vi "Save.vi"(8 "error in (no error)":errorcluster, 9 "new command":string, 10 "Msg in":T1, 11 "FakePressureController in":refnum<class "Tapedrive_ESP301.lvclass">) -> (0 "error out":errorcluster, 1 "Path":path, 2 "Msg out":T1, 3 "FakePressureController out":refnum<class "Tapedrive_ESP301.lvclass">, 4 "new command":string)   [LabVIEW 2011, in "Tapedrive_ESP301.lvclass"]
uses:
  Tapedrive_ESP301.lvclass
  DriverMsg.ctl
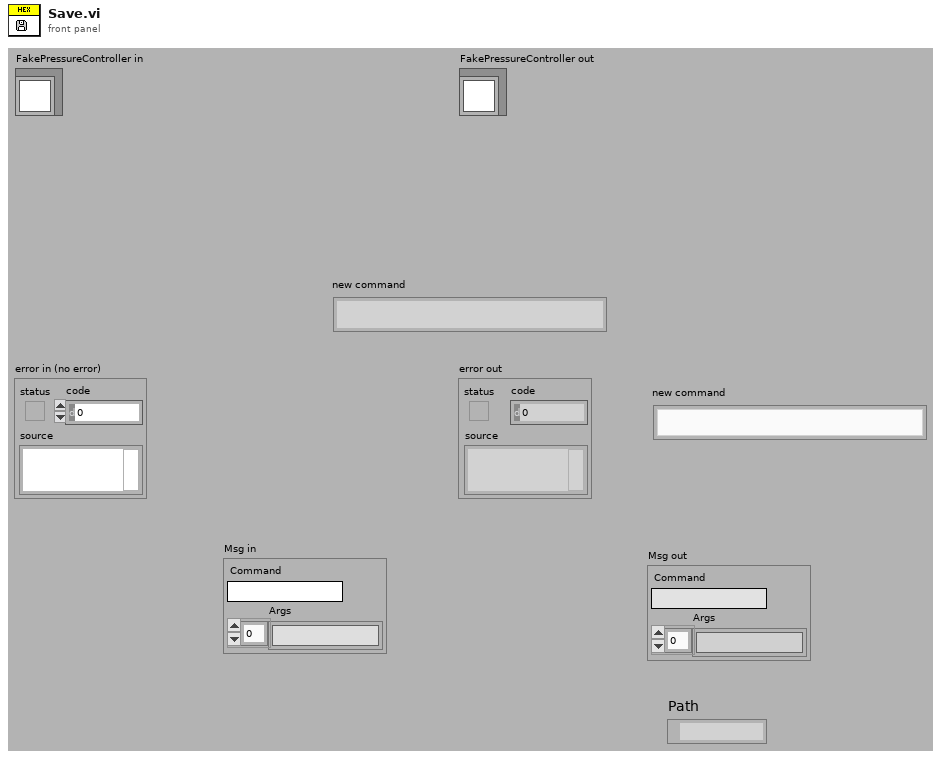
[diagram p1: front panel]
types:
  T1 = typedef "DriverMsg.ctl" = cluster{"Command":string, "Args":string[]}
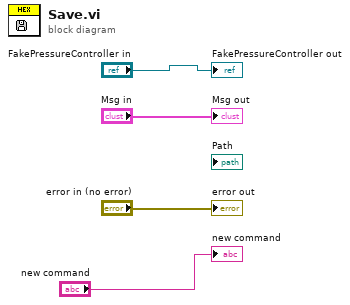
[diagram p0: block diagram]
diagram:
  "error out" <- "error in (no error)"
  "FakePressureController out" <- "FakePressureController in"
  "Msg out" <- "Msg in"
  "new command" <- "new command"
